vi "Get Slave Info.vi"(8 "error in (no error)":errorcluster, 11 "Item Ref in":T1 format="%.0x") -> (0 "error out":errorcluster, 1 "Slave #":u16, 2 "Slave Name":string, 3 "Item Ref out":T1 format="%.0x", 4 "Distributed Clock":bool, 5 "Prepend":bool)   [LabVIEW 2020, in "SEECD System Explorer.lvlib"]
uses:
  SEECD System Explorer.lvlib
  <vilib>/NI VeriStand/Custom Device API/Custom Device Item Ref.ctl
  Shared/Globals/Property Strings.vi
  <vilib>/NI VeriStand/Custom Device API/Get Item Property (Boolean).vi
  <vilib>/NI VeriStand/Custom Device API/Get Item Property (U16).vi
  <vilib>/NI VeriStand/Custom Device API/Custom Device API.lvlib
  Shared/SEECD Shared.lvlib
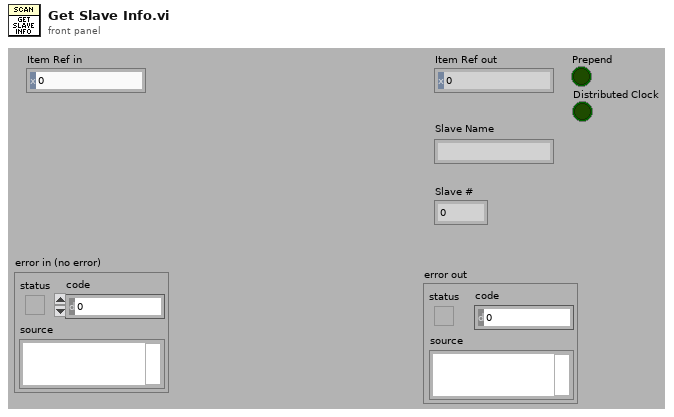
[diagram p1: front panel]
types:
  T1 = typedef "Custom Device API.lvlib/Custom Device Item Ref.ctl" = u64
  T2 = typedef "Custom Device API.lvlib/Custom Device Item Info.ctl" = cluster{"Name":string, "Is Channel":bool, "GUID":string, "Is Waveform":bool}
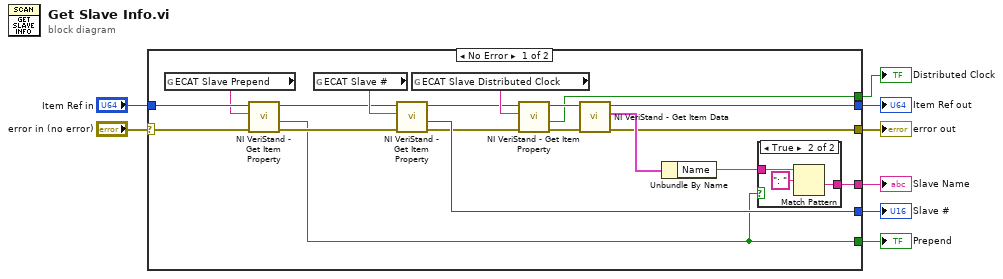
[diagram p0: block diagram]
diagram:
  n1 = case shown="No Error" "error in (no error)" {
    selector: "error in (no error)" -> [w19 w33]
    tunnel: [w23 w33] -> w7
    tunnel: "Item Ref in" -> [w20 w32]
    tunnel: [w24 w32] -> w5
    tunnel: [w22 _] -> w4
    tunnel: [w21 _] -> w3
    tunnel: [w15 _] -> w2
    tunnel: [w9 _] -> w1
    frame No Error {
      n2 = global read "Property Strings.vi" "ECAT Slave Prepend"() -> (w18:string)
      n3 = call-poly <vilib>:"NI VeriStand - Get Item Property.vi"("error in (no error)"=w19, "Property Name"=w18, "Item Ref in"=w20) -> ("error out"=w16:errorcluster, "Value"=w15:bool, "Item Ref out"=w17:T1)  [unwired: 5 in, 1 out]
      n4 = global read "Property Strings.vi" "ECAT Slave #"() -> (w27:string)
      n5 = call-poly <vilib>:"NI VeriStand - Get Item Property.vi"("error in (no error)"=w16, "Property Name"=w27, "Item Ref in"=w17) -> ("error out"=w13:errorcluster, "Value"=w21:u16, "Item Ref out"=w10:T1)  [unwired: 5 in, 1 out]
      n6 = global read "Property Strings.vi" "ECAT Slave Distributed Clock"() -> (w14:string)
      n7 = call-poly <vilib>:"NI VeriStand - Get Item Property.vi"("error in (no error)"=w13, "Property Name"=w14, "Item Ref in"=w10) -> ("error out"=w12:errorcluster, "Value"=w9:bool, "Item Ref out"=w11:T1)  [unwired: 5 in, 1 out]
      n8 = call <vilib>:"NI VeriStand - Get Item Data.vi"("error in (no error)"=w12, "Item Ref in"=w11) -> ("error out"=w23:errorcluster, "Item Info"=w25:T2, "Item Ref out"=w24:T1)  [unwired: 7 out]
      n9 = Unbundle By Name(w25) -> ("Name"=w26:string)
      n10 = case shown="True" w15 {
        tunnel: w26 -> [w28 w30]
        tunnel: [w28 w29] -> w22
        frame False {
        }
        frame True {
          n11 = Match Pattern(string=w30, regular expression=": " ("search string/char (-)")) -> (after substring=w29:string)  [unwired: 1 in, 3 out]
        }
      }
    }
    frame Error {
    }
  }
  "error out" <- w7
  "Item Ref out" <- w5
  "Slave #" <- w3
  "Slave Name" <- w4
  "Prepend" <- w2
  "Distributed Clock" <- w1
